vi "Open Settings Dialog.vi"(8 "error in (no error)":errorcluster, 11 "HIJ Vision Camera App in":refnum<class "HIJ Vision Camera App.lvclass">) -> (0 "error out":errorcluster, 3 "HIJ Vision Camera App out":refnum<class "HIJ Vision Camera App.lvclass">)   [LabVIEW 2020, in "HIJ Vision Camera App.lvlib" / "HIJ Vision Camera App.lvclass"]
uses:
  HIJ Vision Camera App.lvclass
  C:/Users/AlexK/work/LabVIEW Programme/POLARIS CAM Log Abw und E/Submodules/HIJ Vision/Application Base Actors/HIJ Vision Application/HIJ Vision Application/HIJ Vision Application.lvclass
  C:/Program Files (x86)/National Instruments/LabVIEW 2020/vi.lib/ActorFramework/Actor/Actor.lvclass
  HIJ Vision Camera App.lvclass/HIJ Vision Camera App.ctl
  HIJ Vision Camera App Dialog/HIJ Vision Camera App Dialog/HIJ Vision Camera App Dialog.lvclass
  HIJ Vision Application/HIJ Vision Application/HIJ Vision Application.lvclass/HIJ Vision Application.ctl
  HIJ Vision Camera App Dialog/HIJ Vision Camera App Dialog/HIJ Vision Camera App Dialog.lvclass/HIJ Vision Camera App Dialog.ctl
  <vilib>/ActorFramework/Message Enqueuer/Message Enqueuer.lvclass/Message Enqueuer.ctl
  Read Prefix.vi
  HIJ Vision Application/HIJ Vision Application/Read WorkDir.vi
  Read Camera Name.vi
  HIJ Vision Camera App Dialog/HIJ Vision Camera App Dialog/Write Prefix.vi
  HIJ Vision Camera App Dialog/HIJ Vision Camera App Dialog/Write WorkDir.vi
  HIJ Vision Camera App Dialog/HIJ Vision Camera App Dialog/Write Camera Name.vi
  <vilib>/ActorFramework/Message Enqueuer/Enqueue.vi
  Viewable Actor/ViewableActor Messages/Open Front Panel Msg/Open Front Panel Msg.lvclass
  C:/Program Files (x86)/National Instruments/LabVIEW 2020/vi.lib/ActorFramework/Message/Message.lvclass
  <vilib>/ActorFramework/Message Priority Queue/Priority Enqueue.vi
  <vilib>/ActorFramework/Message Enqueuer/Message Enqueuer.lvclass
  <vilib>/ActorFramework/Actor/Actor.lvclass
  Viewable Actor/ViewableActor.lvlib
  C:/Users/AlexK/work/LabVIEW Programme/POLARIS CAM Log Abw und E/Submodules/Viewable Actor/ViewableActor/ViewableActor.lvclass
  C:/Users/AlexK/work/LabVIEW Programme/POLARIS CAM Log Abw und E/Submodules/HIJ Vision/Application Base Actors/HIJ Vision Camera App Dialog/HIJ Vision Camera App Dialog/HIJ Vision Camera App Dialog.lvclass
  C:/Users/AlexK/work/LabVIEW Programme/POLARIS CAM Log Abw und E/Submodules/HIJ Vision/Analyze/Analyze Actor/IAnalysis/IAnalysis.lvclass
  C:/Users/AlexK/work/LabVIEW Programme/POLARIS CAM Log Abw und E/Submodules/HIJ Vision/Application Base Actors/HIJ Vision Camera App/HIJ Vision Camera App/HIJ Vision Camera App.lvclass
  C:/Users/AlexK/work/LabVIEW Programme/POLARIS CAM Log Abw und E/Submodules/HIJ Vision/Camera Actors/Camera Actor/ICamera/ICamera.lvclass
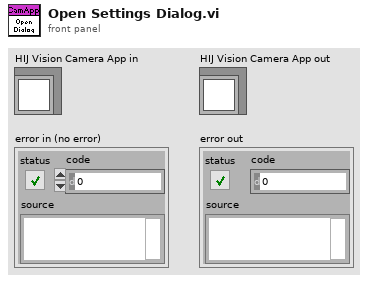
[diagram p1: front panel]
types:
  T1 = typedef "LVPositionTypeDef.ctl" = cluster{"Left":i32, "Top":i32}
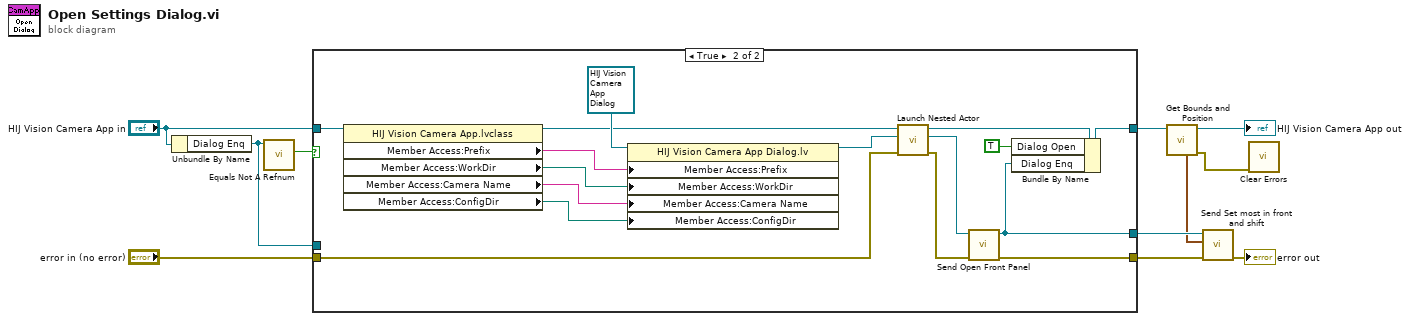
[diagram p0: block diagram]
diagram:
  n1 = Unbundle By Name("HIJ Vision Camera App in") -> ("Dialog Enq"=w4:refnum<class "Message Enqueuer.lvclass">)
  n2 = call <vilib>:"Equals Not A Refnum.vi"("Message Enqueuer"=w4) -> ("Not a refnum?"=w7:bool)  [unwired: 10 in]
  n3 = case shown="True" w7 {
    tunnel: [w14 w24] -> w8
    tunnel: "HIJ Vision Camera App in" -> [w14 w29]
    tunnel: "error in (no error)" -> [w13 w27]
    tunnel: [w13 w25] -> w11
    tunnel: [w12 w21] -> w5
    tunnel: w4 -> [w12 _]
    frame False {
    }
    frame True {
      n4 = property class="HIJ Vision Camera App.lvclass"(reference=w29) -> (reference out=w19:refnum<class "HIJ Vision Camera App.lvclass">, "Member Access:Prefix"=w18:string, "Member Access:WorkDir"=w17:path, "Member Access:Camera Name"=w16:string, "Member Access:ConfigDir"=w15:path)  [unwired: 1 in, 1 out]
      n5 = property class="HIJ Vision Camera App Dialog.lv"(reference=refnum<class "HIJ Vision Camera App Dialog.lvclass"> refnum, "Member Access:Prefix"=w18, "Member Access:WorkDir"=w17, "Member Access:Camera Name"=w16, "Member Access:ConfigDir"=w15) -> (reference out=w20:refnum<class "HIJ Vision Camera App Dialog.lvclass">)  [unwired: 1 in, 1 out]
      n6 = call <vilib>:"Launch Nested Actor.vi"("error in (no error)"=w27, "Nested Actor"=w20, "Caller Actor in"=w19) -> ("error out"=w26:errorcluster, "Nested Actor's Enqueuer"=w23:refnum<class "Message Enqueuer.lvclass">, "Caller Actor out"=w28:refnum<class "HIJ Vision Camera App.lvclass">)  [unwired: 6 in]
      n7 = call "Send Open Front Panel.vi"("error in (no error)"=w26, "Message Enqueuer"=w23) -> ("error out"=w25:errorcluster, "Message Enqueuer out"=w21:refnum<class "Message Enqueuer.lvclass">)  [unwired: 8 in]
      n8 = Bundle By Name(cluster=w28, "Dialog Open"=TRUE, "Dialog Enq"=w21) -> (w24:refnum<class "HIJ Vision Camera App.lvclass">)
    }
  }
  n9 = call-dynamic "Get Bounds and Position.vi"("ViewableActor in"=w8) -> ("error out"=w1:errorcluster, "ViewableActor out"=→"HIJ Vision Camera App out":refnum<class "HIJ Vision Camera App.lvclass">, "Panel Position"=w2:T1)  [unwired: 6 in, 2 out]
  n10 = call "Send Set most in front and shift.vi"("error in (no error)"=w11, "top left point"=w2, "Message Enqueuer in"=w5) -> ("error out"=→"error out":errorcluster)  [unwired: 8 in]
  n11 = call <vilib>:"Clear Errors.vi"("error in (no error)"=w1) -> ()  [unwired: 5 in, 2 out]
